vi "MH_Init.vi"(8 "error in (no error)":errorcluster, 10 "Mode":T2 items=["HIST"=0, "T2"=2, "T3"=3], 11 "Multiharp in":refnum<class "Multiharp.lvclass">) -> (0 "error out":errorcluster, 3 "Multiharp out":refnum<class "Multiharp.lvclass">)   [LabVIEW 2023, in "Multiharp.lvlib" / "Multiharp.lvclass"]
uses:
  Multiharp.lvclass
  Multiharp.lvclass/Multiharp.ctl
  MultiharpComm Messages/MH_InitDone Msg/MH_InitDone Msg.lvclass
  <vilib>/ActorFramework/Actor/Actor.lvclass
  _lib/PQ/MultiHarp/MH_RefSource.ctl
  _lib/PQ/MultiHarp/MH_MeasMode.ctl
  _lib/PQ/MultiHarp/MH_InitInfo.ctl
  typedefs/typedefs.lvlib
panel:
  in  "event data":cluster{"Init":bool, "nchannels":i32}
  in  "MH Init Done":cluster{"DevIdx":i32, "Init Info":T1}
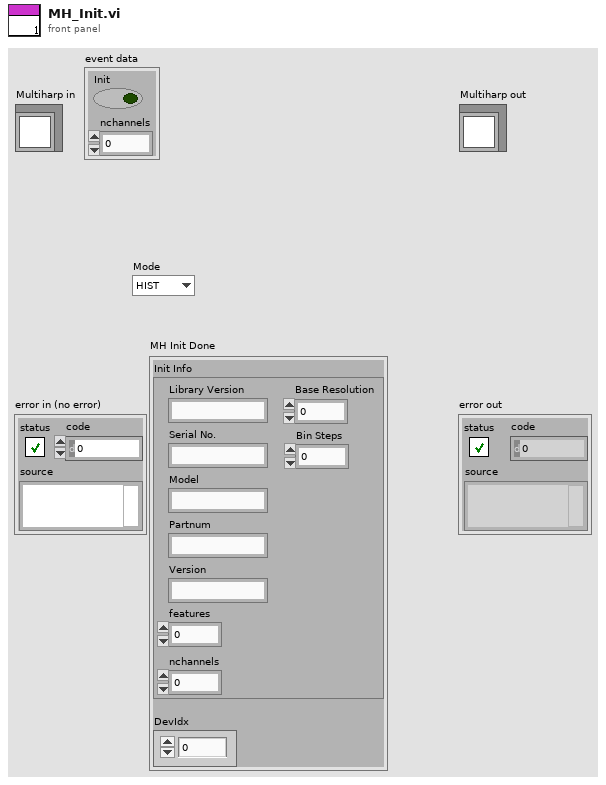
[diagram p1: front panel]
types:
  T1 = typedef "typedefs.lvlib/MH_InitInfo.ctl" = cluster{"Library Version":string, "Serial No.":string, "Model":string, "Partnum":string, "Version":string, "features":i32, "nchannels":i32, "Base Resolution":dbl, "Bin Steps":i32}
  T2 = typedef "MH_MeasMode.ctl" = i32
  T3 = typedef "MH_RefSource.ctl" = enum16{"INTERNAL", "EXTERNAL_10MHZ", "WR_MASTER_GENERIC", "WR_SLAVE_GENERIC", "WR_GRANDM_GENERIC", "EXTN_GPS_PPS", "EXTN_GPS_PPS_UART", "WR_MASTER_MHARP", "WR_SLAVE_MHARP", "WR_GRANDM_MHARP"}
  T4 = typedef "typedefs.lvlib/InstrumentData.ctl" = cluster{"Instr Error":errorcluster, "Address":cluster{"address type":enum16{"VISA", "Index"}, "Address":string, "instrument type":T5}, "CurrentState":cluster{"Initialized":bool, "Connected":bool, "Running":bool, "Error":bool}}
  T5 = typedef "typedefs.lvlib/instrumentType.ctl" = enum16{"Spectrometer", "Camera", "Stepper", "Piezo", "SLM"}
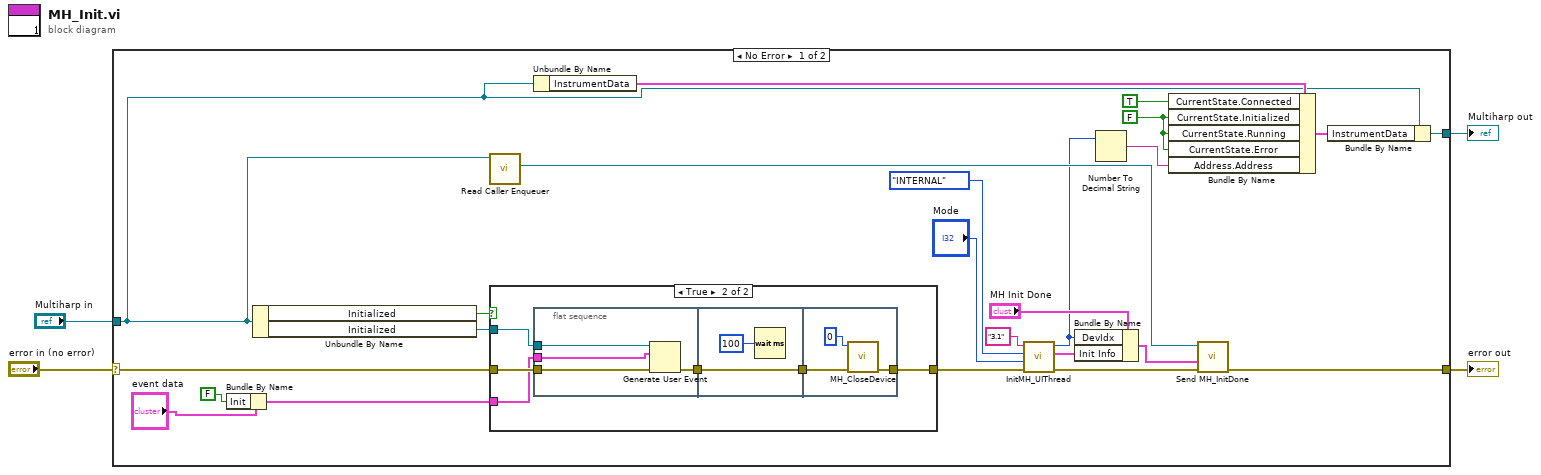
[diagram p0: block diagram]
diagram:
  n1 = case shown="No Error" "error in (no error)" {
    selector: "error in (no error)" -> [w15 w46]
    tunnel: [w18 w46] -> w3
    tunnel: [w9 w45] -> w1
    tunnel: "Multiharp in" -> [w5 w45]
    frame No Error {
      w22 = FALSE ("CurrentState.Connected")
      n2 = Bundle By Name(cluster="event data", "Init"=FALSE) -> (w14:cluster{"Init":bool, "nchannels":i32})
      n3 = Unbundle By Name(w5) -> ("Initialized"=w20:bool, "Initialized"=w12:refnum<user-event>)
      n4 = call <vilib>:"Read Caller Enqueuer.vi"("Actor"=w5) -> ("Caller Enqueuer"=w21:refnum<class "Message Enqueuer.lvclass">)  [unwired: 10 in]
      n5 = case shown="True" w20 {
        tunnel: [w29 w35] -> w19
        tunnel: w12 -> [_ w32]
        tunnel: w15 -> [w29 w31]
        tunnel: w14 -> [_ w30]
        frame False {
        }
        frame True {
          n6 = flat-sequence {
            tunnel: [w37] -> w33
            tunnel: w32 -> [w39]
            tunnel: w31 -> [w38]
            tunnel: w30 -> [w36]
            tunnel: [w41] -> w34
            tunnel: w33 -> [w41]
            tunnel: [w43] -> w35
            tunnel: w34 -> [w42]
            frame #0 {
              n7 = Generate User Event(user event=w39, event data cluster=w36, error in=w38) -> (error out=w37:errorcluster)  [unwired: 1 in, 1 out]
            }
            frame #1 {
              n8 = Wait (ms)(milliseconds to wait=u32 100) -> ()  [unwired: 1 out]
            }
            frame #2 {
              n9 = call "MH_CloseDevice.vi"("error in (no error)"=w42, "devidx"=0) -> ("error out"=w43:errorcluster)  [unwired: 8 in, 1 out]
            }
          }
        }
      }
      n10 = Unbundle By Name(w5) -> ("InstrumentData"=w10:T4)
      n11 = call "InitMH_UIThread.vi"("error in (no error)"=w19, "Mode"="Mode", "refsource"=MH_RefSource."INTERNAL", "Library Version"="3.1") -> ("error out"=w11:errorcluster, "Init Info"=w25:T1, "DevIdx"=w17:i32)  [unwired: 5 in]
      n12 = Bundle By Name(cluster="MH Init Done", "DevIdx"=w17, "Init Info"=w25) -> (w24:cluster{"DevIdx":i32, "Init Info":T1})
      n13 = Number To Decimal String(number=w17) -> (decimal integer string=w16:string)  [unwired: 1 in]
      n14 = Bundle By Name(cluster=w10, "CurrentState.Connected"=TRUE, "CurrentState.Initialized"=w22, "CurrentState.Running"=w22, "CurrentState.Error"=w22, "Address.Address"=w16) -> (w7:T4)
      n15 = call "Send MH_InitDone.vi"("error in (no error)"=w11, "MH Init Done"=w24, "Message Enqueuer"=w21) -> ("error out"=w18:errorcluster)  [unwired: 7 in, 1 out]
      n16 = Bundle By Name(cluster=w5, "InstrumentData"=w7) -> (w9:refnum<class "Multiharp.lvclass">)
    }
    frame Error {
    }
  }
  "error out" <- w3
  "Multiharp out" <- w1
